vi "uncoverspace.vi"(6 "input array":i8[][][](array[numeric]), 9 "j":i32, 10 "i":i32, 11 "k":i32) -> (4 "win?":i32, 7 "output array":i8[][][](array[numeric]), 8 "win2":i32)   [LabVIEW 2025]
uses:
  c_code/uncoverspace_lock252564.dll
panel:
  out "error out":errorcluster
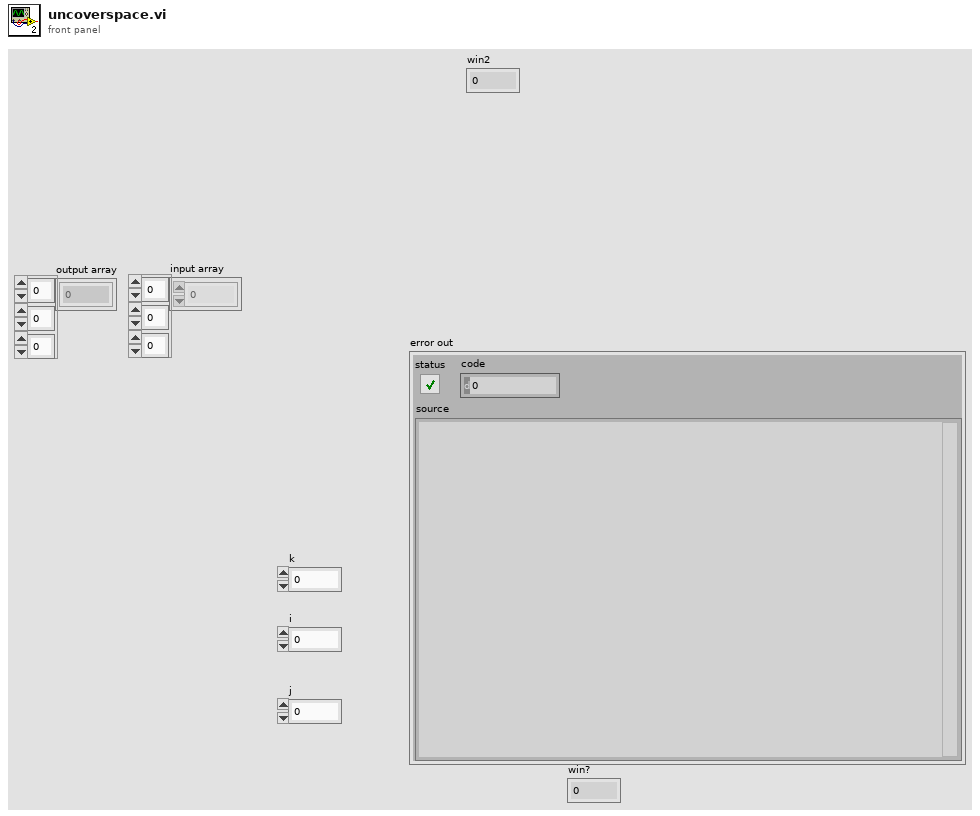
[diagram p1: front panel]
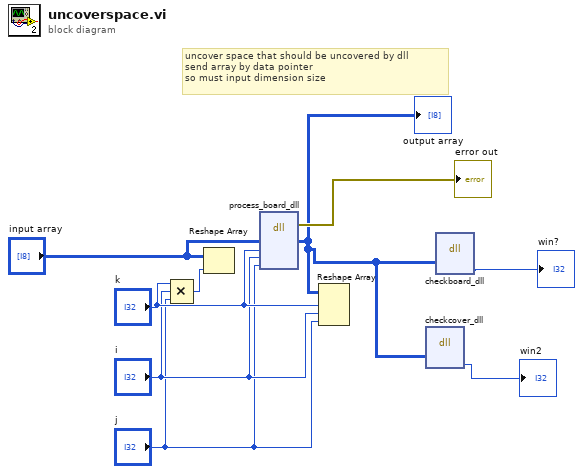
[diagram p0: block diagram]
diagram:
  # "uncover space that should be uncovered by dll\nsend array by data pointer\nso must input dimension size"
  n1 = Compound Arithmetic op=MULTIPLY("k", "i", "j") -> (w8:i32)
  n2 = Reshape Array("input array", w8) -> ()  [unwired: 1 out]
  n3 = dll-call lib="C:/Users/daimapi/Desktop/project/minesweeper/c_code/uncoverspace_lock252564.dll" fn="process_board_dll"("arg1"="input array", "z"="k", "y"="i", "x"="j") -> (error out=→"error out":errorcluster, "arg1"=w2:i8[][][])  [unwired: 7 in, 1 out]
  "output array" <- w2
  n4 = Reshape Array(w2, "k", "i", "j") -> ()  [unwired: 1 out]
  n5 = dll-call lib="C:/Users/daimapi/Desktop/project/minesweeper/c_code/uncoverspace_lock252564.dll" fn="checkcover_dll"("arg1"=w2) -> ("win?"=→"win2":i32)  [unwired: 6 in, 2 out]
  n6 = dll-call lib="C:/Users/daimapi/Desktop/project/minesweeper/c_code/uncoverspace_lock252564.dll" fn="checkboard_dll"("arg1"=w2) -> ("win?"=→"win?":i32)  [unwired: 6 in, 2 out]
